vi "Test Thermocouple.vi"() -> ()   [LabVIEW 2020]
uses:
  <vilib>/DAQmx/create/channels.llb/DAQmx Create Channel (AI-Temperature-Thermocouple).vi
  <vilib>/DAQmx/read.llb/DAQmx Read (Analog DBL 1Chan 1Samp).vi
panel:
  out "Waveform Chart":dbl(graph)
  in  "stop":bool
  in  "cjc value":dbl=25.0 format="%0.2f"
  in  "cjc source":i32(ring)=10116 items=["Built-In"=10200, "Constant Value"=10116, "Channel"=10113]
  in  "minimum value":dbl format="%0.2f"
  in  "maximum value":dbl=100.0 format="%0.2f"
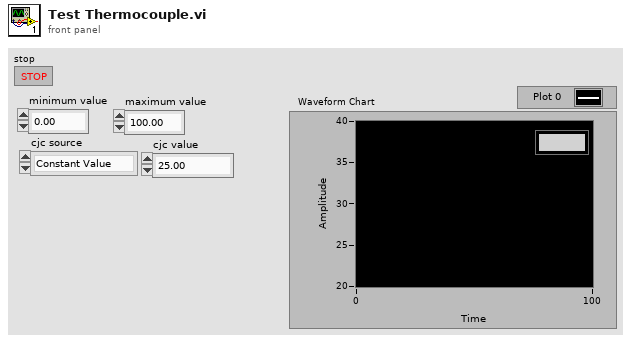
[diagram p1: front panel]
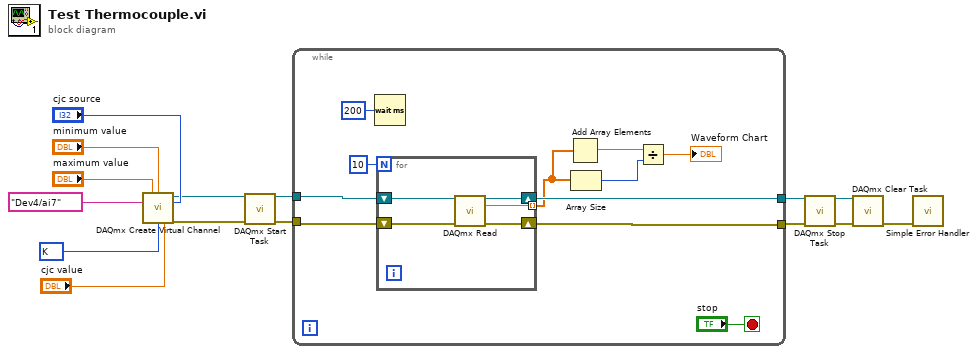
[diagram p0: block diagram]
diagram:
  w11 = 10073 items=["J"=10072, "K"=10073, "N"=10077, "R"=10082, "S"=10085, "T"=10086, "B"=10047, "E"=10055] ("thermocouple type")
  n1 = call-poly <vilib>:"DAQmx Create Virtual Channel.vi"("maximum value"="maximum value", "minimum value"="minimum value", "physical channels"=tag "Dev4/ai7", "cjc source"="cjc source", "thermocouple type"=w11, "cjc value"="cjc value") -> ("task out"=w8:refnum<k21>, "error out"=w9:errorcluster)  [unwired: 8 in]
  n2 = call <vilib>:"DAQmx Start Task.vi"("task/channels in"=w8, "error in"=w9) -> ("task out"=w6:refnum<k21>, "error out"=w7:errorcluster)  [unwired: 12 in]
  n3 = while {
    tunnel: w7 -> [w26]
    tunnel: w6 -> [w25]
    tunnel: [w23] -> w5
    tunnel: [w22] -> w4
    stop <- "stop" stop-if-true
    n4 = Wait (ms)(milliseconds to wait=u32 200) -> ()  [unwired: 1 out]
    n5 = for {
      N: 10 -> [_]
      shift-right: [w29] -> w23
      shift-left: w26 -> [w31]
      shift-right: [w28] -> w22
      shift-left: w25 -> [w30]
      tunnel: [w27] -> w16 mode=indexing
      n6 = call-poly <vilib>:"DAQmx Read.vi"("task/channels in"=w30, "error in"=w31) -> ("task out"=w28:refnum<k21>, "data"=w27:dbl, "error out"=w29:errorcluster)  [unwired: 11 in]
    }
    n7 = Add Array Elements(numeric array=w16) -> (sum=w20:dbl)
    n8 = Array Size(array=w16) -> (size(s)=w19:i32)
    n9 = Divide(x=w20, y=w19) -> (x/y=→"Waveform Chart":dbl)
  }
  n10 = call <vilib>:"DAQmx Stop Task.vi"("task/channels in"=w4, "error in"=w5) -> ("task out"=w2:refnum<k21>, "error out"=w3:errorcluster)  [unwired: 12 in]
  n11 = call <vilib>:"DAQmx Clear Task.vi"("task in"=w2, "error in"=w3) -> ("error out"=w1:errorcluster)  [unwired: 13 in]
  n12 = call <vilib>:"Simple Error Handler.vi"("error in (no error)"=w1) -> ()  [unwired: 4 in, 5 out]
